vi "fake_read_horizontal line.vi"(1 "line counter":u16) -> (0 "input cluster":T1)   [LabVIEW 2010]
uses:
  common_typedefs/channels_cluster.ctl
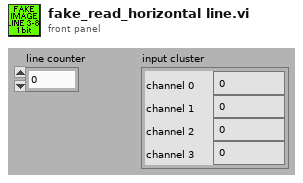
[diagram p1: front panel]
types:
  T1 = typedef "channels_cluster.ctl" = cluster{"channel 0":u32, "channel 1":u32, "channel 2":u32, "channel 3":u32}
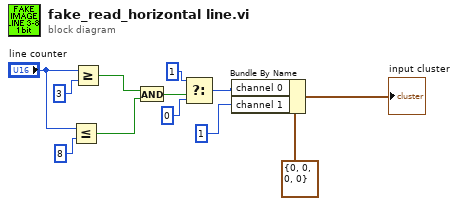
[diagram p0: block diagram]
diagram:
  n1 = Less Or Equal?(x="line counter", y=u16 8) -> (x <= y?=w1:bool)
  n2 = Greater Or Equal?(x="line counter", y=u16 3) -> (x >= y?=w6:bool)
  n3 = And(x=w6, y=w1) -> (x .and. y?=w7:bool)
  n4 = Select(t=u16 1 ("y"), s=w7, f=u16 0) -> (s? t:f=w10:u16)
  n5 = Bundle By Name(cluster=T1 {"channel 0"=0, "channel 1"=0, "channel 2"=0, "channel 3"=0} ("input cluster"), "channel 0"=w10, "channel 1"=u16 1 ("f")) -> (→"input cluster":T1)
